vi "_TangoSubscribeAttributeConfigEvent.vi"(1 "error in":errorcluster, 2 "attribute name":string, 3 "device name":string, 4 "attribute config event ref":T1) -> (0 "error out":errorcluster)   [LabVIEW 2014, in "tango.lvlib"]
uses:
  tango.lvlib
  Common VIs/Typedefs/_AttributeConfigEventRef.ctl
  Common VIs/Typedefs/_AttributeInfo_t.ctl
  Common VIs/Typedefs/_AttributeAccess_t.ctl
  Common VIs/Typedefs/_AttributeFormat_t.ctl
  Common VIs/Typedefs/_TangoDataType_t.ctl
  Common VIs/Typedefs/_AttributeLevel_t.ctl
  Private VIs/Events/_EventType.ctl
  tango_binding.so
panel:
  out "evt identifier":i32
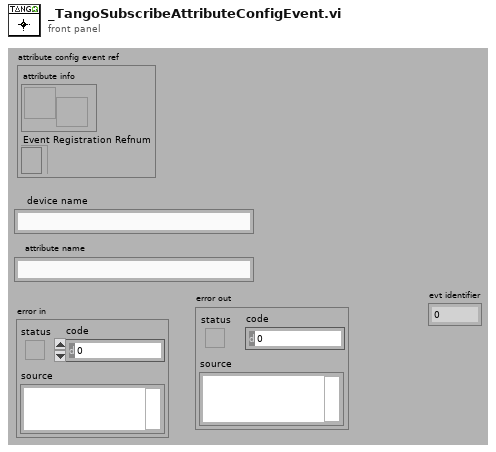
[diagram p1: front panel]
types:
  T1 = typedef "tango.lvlib/_AttributeConfigEventRef.ctl" = cluster{"attribute info":refnum<user-event>, "Event Registration Refnum":refnum<event-registration>}
  T2 = typedef "tango.lvlib/_EventType.ctl" = enum32{"CHANGE_EVENT", "DEPRECATED_QUALITY_EVENT", "PERIODIC_EVENT", "ARCHIVE_EVENT", "USER_EVENT", "ATTRIBUTE_CONF_EVENT", "DATA_READY_EVENT", "INTERFACE_CHANGE_EVENT", "UNKNOWN_EVENT"}
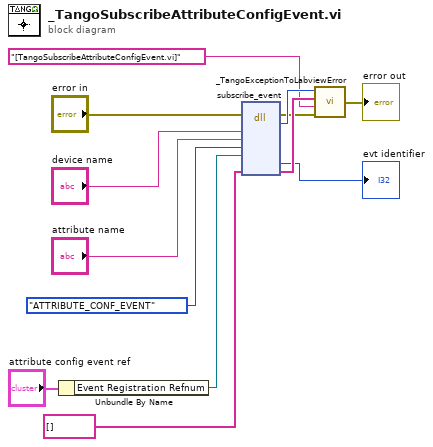
[diagram p0: block diagram]
diagram:
  n1 = Unbundle By Name("attribute config event ref") -> ("Event Registration Refnum"=w4:refnum<event-registration>)
  n2 = dll-call lib="tango_binding.*" fn="subscribe_event"(error in="error in", "dev_name"="device name", "attr_name"="attribute name", "evt_type"=_EventType."ATTRIBUTE_CONF_EVENT", "evt_ref"=w4, "error_stack_"=string[] [] ("subscribe error stack")) -> (error out=w7:errorcluster, "return type"=w10:i32, "evt_identifier"=→"evt identifier":i32, "error_stack_"=w9:string[])  [unwired: 7 in, 1 out]
  n3 = call "_TangoExceptionToLabviewError.vi"("error in"=w7, "location"="[TangoSubscribeAttributeConfigEvent.vi]", "error stack"=w9, "error code"=w10) -> ("error out"=→"error out":errorcluster)
